vi "Klaster_001_PH.vi"() -> ()   [LabVIEW 2021]
panel:
  out "Cluster 2":T1={"Array"=[2020, 2020, 2020, 2020, 2020], "Boolean"=FALSE, "String"="pierwszy cluster"}
  in  "Cluster":T1={"Array"=[2020, 2020, 2020, 2020, 2020], "Boolean"=FALSE, "String"="pierwszy cluster"}
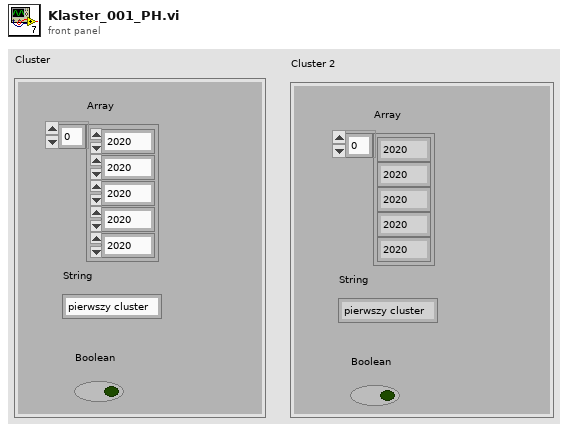
[diagram p1: front panel]
types:
  T1 = cluster{"Array":i16[], "Boolean":bool, "String":string}
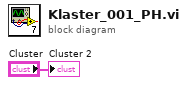
[diagram p0: block diagram]
diagram:
  "Cluster 2" <- "Cluster"
